vi "REPORT_OPRTN_prepare_archivisation_info.vi"(11 "records_from_SQL":string[][](array[string])) -> (2 "archivisation_description":string[][](array[string]), 3 "archivisation_info":string[][](array[string]))   [LabVIEW 2019]
uses:
  FGV/SQL_connection/FGV_CLIENT_SQL_connection.ctl
  <userlib>/_OpenG.lib/array/array.llb/Reorder 2D Array2 (String)__ogtk.vi
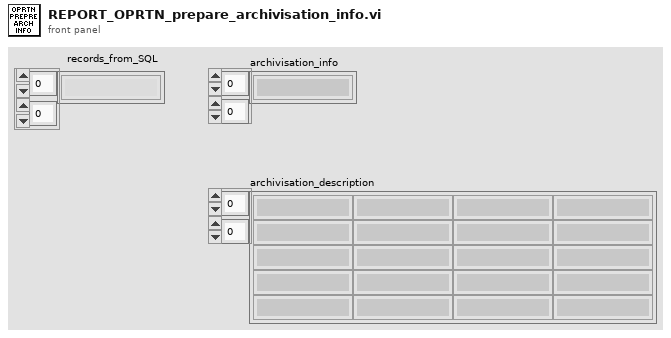
[diagram p1: front panel]
types:
  T1 = typedef "FGV_CLIENT_SQL_connection.ctl" = enum16{"initialize", "connect", "read_tables", "read_columns", "SELECT", "INSERT", "UPDATE", "DELETE", "EXEC + headers", "EXEC", "TRANSACTION", "connection_active?", "disconnect"}
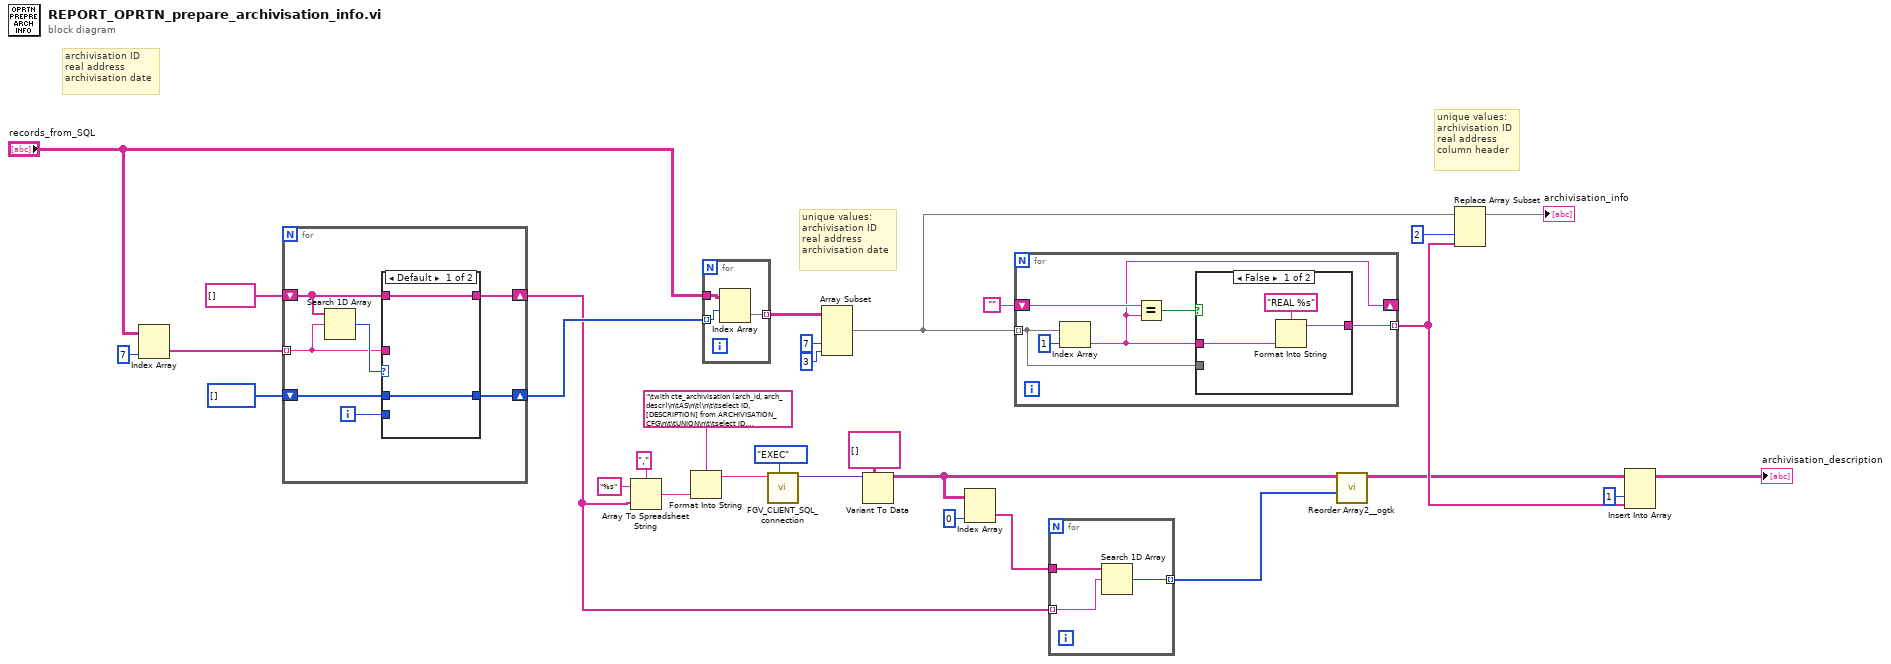
[diagram p0: block diagram]
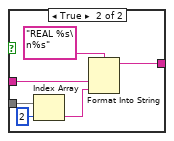
[diagram p2: hidden frame]
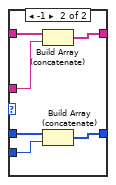
[diagram p3: hidden frame]
diagram:
  # "unique values:\narchivisation ID\nreal address\ncolumn header"
  # "unique values:\narchivisation ID\nreal address\narchivisation date"
  # "archivisation ID\nreal address\narchivisation date"
  n1 = Index Array(array="records_from_SQL", index (col)=7 ("disabled index (col)")) -> (element=w26:string[])  [unwired: 1 in]
  n2 = for {
    tunnel: w26 -> [w36] mode=indexing
    shift-right: [w35] -> w1
    shift-left: string[] [] -> [w34]
    shift-right: [w32] -> w28
    shift-left: i32[] [] -> [w31]
    i -> [w33]
    n3 = Search 1D Array(1D array=w34, element=w36) -> (index of element=w37:i32)  [unwired: 1 in]
    n4 = case shown="Default" w37 {
      tunnel: w36 -> [_ w45]
      tunnel: [w39 w43] -> w35
      tunnel: w34 -> [w39 w44]
      tunnel: w33 -> [_ w40]
      tunnel: [w38 w41] -> w32
      tunnel: w31 -> [w38 w42]
      frame Default {
      }
      frame -1 {
        n5 = Build Array (concatenate)(w44, w45) -> (w43:string[])
        n6 = Build Array (concatenate)(w42, w40) -> (w41:i32[])
      }
    }
  }
  n7 = Array To Spreadsheet String(delimiter (Tab)=",", array=w1, 3:"%s" ("format string")) -> (spreadsheet string=w18:string)
  n8 = Format Into String(format string="\twith cte_archivisation (arch_id, arch_descr)\n\tAS\n\t(\n\t\tselect ID, [DESCRIPTION] from ARCHIVISATION_CFG\n\t\tUNION\n\t\tselect ID, [DESCRIPTION] from ARCHIVISATION_CFG_HISTORY\n\t)\n\n\tSELECT arch_id, arch_descr\n\tFROM cte_archivisation\n\tWHERE arch_id IN (%s)\nORDER BY arch_id", w18) -> (resulting string=w16:string)  [unwired: 2 in, 1 out]
  n9 = for {
    tunnel: "records_from_SQL" -> [w48]
    tunnel: [w47] -> w24 mode=indexing
    tunnel: w28 -> [w46] mode=indexing
    n10 = Index Array(array=w48, index (row)=w46) -> (element=w47:string[])  [unwired: 1 in]
  }
  n11 = call "FGV_CLIENT_SQL_connection.vi"("options"=FGV_CLIENT_SQL_connection."EXEC", "SQL_statement"=w16) -> ("SQL_result"=w15:variant)  [unwired: 5 in, 4 out]
  n12 = Array Subset(array=w24, index (col)=7 ("index"), length (col)=3 ("length")) -> (w12:string[][])  [unwired: 2 in]
  n13 = Variant To Data(type=string[][] [], Variant=w15) -> (data=w5:string[][])  [unwired: 1 in, 1 out]
  n14 = Index Array(array=w5, index (col)=0 ("disabled index (col)")) -> (element=w2:string[])  [unwired: 1 in]
  n15 = for {
    tunnel: w12 -> [w49] mode=indexing
    shift-right: [w51] -> _
    shift-left: "" -> [w52]
    tunnel: [w50] -> w9 mode=indexing
    n16 = Index Array(array=w49, index=1) -> (element=w51:string)
    n17 = Equal?(x=w52, y=w51) -> (x = y?=w53:bool)
    n18 = case shown="False" w53 {
      tunnel: w51 -> [w57 w63]
      tunnel: [w56 w62] -> w50
      tunnel: w49 -> [_ w60]
      frame False {
        n19 = Format Into String(format string="REAL %s", w57) -> (resulting string=w56:string)  [unwired: 2 in, 1 out]
      }
      frame True {
        n20 = Index Array(array=w60, index=2) -> (element=w58:string)
        n21 = Format Into String(format string="REAL %s\n%s", w63, w58) -> (resulting string=w62:string)  [unwired: 2 in, 1 out]
      }
    }
  }
  n22 = for {
    tunnel: w1 -> [w64] mode=indexing
    tunnel: w2 -> [w65]
    tunnel: [w66] -> w3 mode=indexing
    n23 = Search 1D Array(1D array=w65, element=w64) -> (index of element=w66:i32)  [unwired: 1 in]
  }
  n24 = call-poly <userlib>:"Reorder Array2__ogtk.vi"("indices"=w3, "array"=w5) -> ("reordered array"=w6:string[][])  [unwired: 9 in]
  n25 = Replace Array Subset(array=w12, new element=w9, index (col)=2 ("disabled index (col)")) -> (→"archivisation_info":string[][])  [unwired: 1 in]
  n26 = Insert Into Array(array=w6, index (col)=1 ("disabled index (col)"), new element=w9) -> (→"archivisation_description":string[][])  [unwired: 1 in]
